vi "Get_Speeds_for_Displac_in_Trees_or_Frames-2.vi"(4 "error IN":errorcluster, 7 "[IN] Displacements in Frame-to-\nFrame Manner or in Tracks (Trees)":dbl[][](array[numeric])) -> (0 "error OUT":errorcluster, 3 "[OUT] Velocities\nin (pixel/frame)":dbl[](array[numeric]))   [LabVIEW 2013]
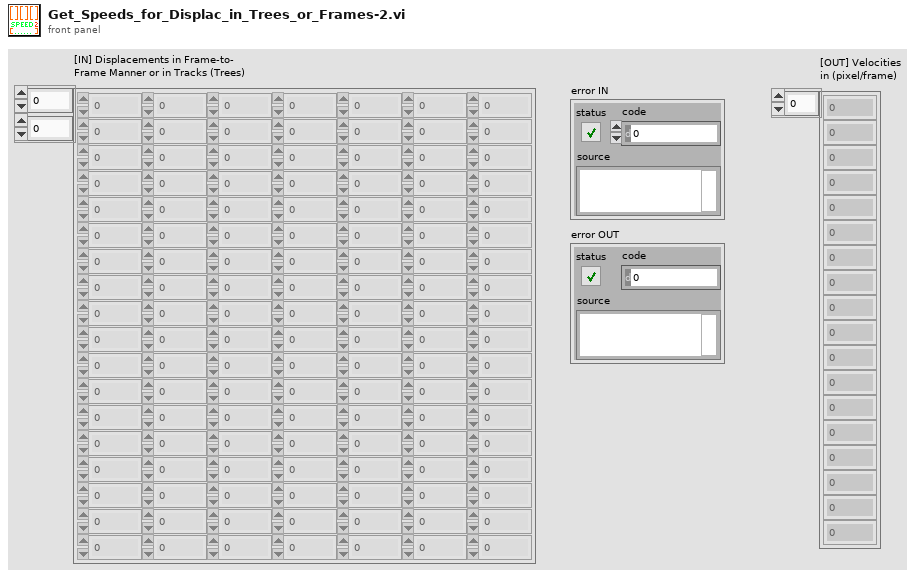
[diagram p1: front panel]
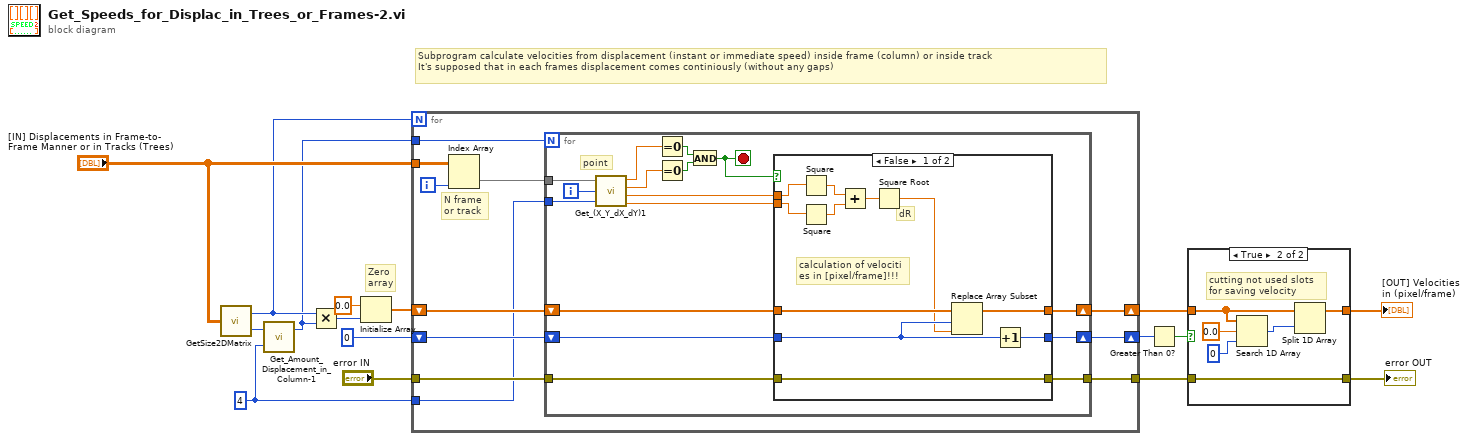
[diagram p0: block diagram]
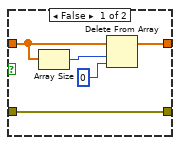
[diagram p2: hidden frame]
diagram:
  w5 = 4 ("y")
  # "Subprogram calculate velocities from displacement (instant or immediate speed) inside frame (column) or inside track\nIt's supposed that in each frames displacement comes continiously (without any gaps)"
  # "Zero\narray"
  n1 = call "GetSize2DMatrix.vi"("Array IN (2D)"="[IN] Displacements in Frame-to-\nFrame Manner or in Tracks (Trees)") -> ("# Cols"=w7:i32, "# Rows"=w6:i32)
  n2 = call "Get_Amount_Displacement_in_Column-1.vi"("multiplier"=w5, "# Rows"=w6) -> ("Displ amount"=w4:i32)  [unwired: 1 out]
  n3 = Multiply(x=w7, y=w4) -> (x*y=w14:i32)
  n4 = Initialize Array(0.0 ("element"), w14) -> (w13:dbl[])
  n5 = for {
    N: w7 -> [_]
    tunnel: "[IN] Displacements in Frame-to-\nFrame Manner or in Tracks (Trees)" -> [w27]
    shift-right: [w21] -> w10
    shift-left: w13 -> [w25]
    tunnel: "error IN" -> [w24]
    shift-right: [w22] -> w9
    shift-left: 0 -> [w23]
    tunnel: [w20] -> w2
    tunnel: w5 -> [w18]
    tunnel: w4 -> [w17]
    i -> [w19]
    # "N frame \nor track"
    n6 = Index Array(array=w27, index (col)=w19) -> (element=w26:dbl[])  [unwired: 1 in]
    n7 = for {
      N: w17 -> [_]
      tunnel: w26 -> [w43]
      tunnel: w18 -> [w41]
      shift-right: [w32] -> w21
      shift-left: w25 -> [w35]
      tunnel: w24 -> [w31]
      shift-right: [w33] -> w22
      shift-left: w23 -> [w34]
      tunnel: [w30] -> w20
      i -> [w42]
      stop <- w38 stop-if-true
      # "point"
      n8 = call "Get_(X_Y_dX_dY)1.vi"("(X,Y,dX,dY)"=w43, "index"=w42, "multiplier"=w41) -> ("X"=w29:dbl, "Y"=w28:dbl, "dX"=w37:dbl, "dY"=w36:dbl)
      n9 = Equal To 0?(x=w29) -> (x = 0?=w39:bool)
      n10 = Equal To 0?(x=w28) -> (x = 0?=w40:bool)
      n11 = And(x=w39, y=w40) -> (x .and. y?=w38:bool)
      n12 = case shown="False" w38 {
        tunnel: w37 -> [w54 _]
        tunnel: w36 -> [w53 _]
        tunnel: w35 -> [w49 w57]
        tunnel: w34 -> [w48 w56]
        tunnel: [w47 w56] -> w33
        tunnel: [w46 w57] -> w32
        tunnel: w31 -> [w45 w55]
        tunnel: [w45 w55] -> w30
        frame False {
          # "calculation of velociti\nes in [pixel/frame]!!!"
          # "dR"
          n13 = Square(x=w54) -> (x^2=w51:dbl)
          n14 = Square(x=w53) -> (x^2=w52:dbl)
          n15 = Add(x=w51, y=w52) -> (x+y=w50:dbl)
          n16 = Square Root(x=w50) -> (sqrt(x)=w44:dbl)
          n17 = Replace Array Subset(array=w49, new element=w44, index=w48) -> (w46:dbl[])
          n18 = Increment(x=w48) -> (x+1=w47:i32)
        }
        frame True {
        }
      }
    }
  }
  n19 = Greater Than 0?(x=w9) -> (x > 0?=w8:bool)
  n20 = case shown="True" w8 {
    tunnel: w10 -> [w60 w65]
    tunnel: [w61 w64] -> w3
    tunnel: w2 -> [w62 w63]
    tunnel: [w62 w63] -> w1
    frame False {
      n21 = Array Size(array=w60) -> (size(s)=w59:i32)
      n22 = Delete From Array(array=w60, length=w59, index=0) -> (array with subset deleted=w61:dbl[])  [unwired: 1 out]
    }
    frame True {
      # "cutting not used slots \nfor saving velocity"
      n23 = Search 1D Array(1D array=w65, element=0.0, start index (0)=0) -> (index of element=w66:i32)
      n24 = Split 1D Array(array=w65, index=w66) -> (first subarray=w64:dbl[])  [unwired: 1 out]
    }
  }
  "error OUT" <- w1
  "[OUT] Velocities\nin (pixel/frame)" <- w3
